vi "Volume ROI entry window.vi"(0 "Coordinates":i32[](array[numeric]), 1 "Do not initialise selector values":bool, 5 "AOLZ Settings":T1, 11 "ZplaneIndex (zero based)":i32, 12 "# of planes":i32) -> (4 "ROIs Info []":T2[](array[typedef]) {"FOV" min=1.0 max=10.0 step=1.0; "Frame Size" min=1.0 max=10.0 step=1.0; "Laser Power" min=1.0 max=10.0 step=0.10000000149011612; "Rel. Resolution" min=1.0 max=10.0 step=1.0; "POI Dwell time" min=1.0 max=10.0 step=0.10000000149011612; "Zoom" min=1.0 max=10.0 step=0.10000000149011612}, 10 "Zoom (out)":dbl=1.0 min=1.0 max=10.0 step=0.10000000149011612, 14 "Cancelled":bool)   [LabVIEW 2020]
uses:
  Typedefs/ROI spec.ctl
  Typedefs/ROI ID Enum.ctl
  ROI Entry screen/Typedefs/ROI Z-stack settings info.ctl
  ROI Entry screen/Typedefs/Volume entry ctrl refs cluster.ctl
  <vilib>/Utility/miscctls.llb/LVPointTypeDef.ctl
  ROI Entry screen/Globals/gl_Volume Entry UI globals.vi
  ROI Entry screen/Globals/gl_ROI Entry UI globals.vi
panel:
  in  "Laser Power (%)":dbl=1.0 min=0.001 max=10.0 step=0.10000000149011612
  in  "Rel. Resolution":dbl=1.0 min=0.001 max=10.0 step=0.10000000149011612
  in  "Dwell Time":dbl=1.0 min=0.001 max=10.0 step=0.10000000149011612
  in  "Z-step (planes)":i32=1 min=1 max=3 step=1
  in  "Dual Rectangle":bool
  in  "Zoom":dbl=1.0 min=0.001 max=10.0 step=0.10000000149011612
  in  "Cancel":bool
  in  "Proceed":bool
  in  "Z-plane 2":u16(ring) caption="Z-plane" items=["Z-plane 1", "Z-plane 2", "Z-plane 3", "Z-plane 4", "Z-plane 5", "Z-plane 6", "Z-plane 7", "Z-plane 8", "Z-plane 9", "Z-plane 10", "Z-plane 11"]
  in  "Z-plane 1":u16(ring) caption="Z-plane" items=["Z-plane 1", "Z-plane 2", "Z-plane 3", "Z-plane 4", "Z-plane 5", "Z-plane 6", "Z-plane 7", "Z-plane 8", "Z-plane 9", "Z-plane 10", "Z-plane 11"]
  in  "Volume":bool
  # "To specify a volume from the drawn rectangle, tick the Volume box and select the z-planes between which the volume should be generated.\n \nTo draw two rectangles at precisely the same XY position but on different z-levels, tick the \"Dual Rectangle\" box."
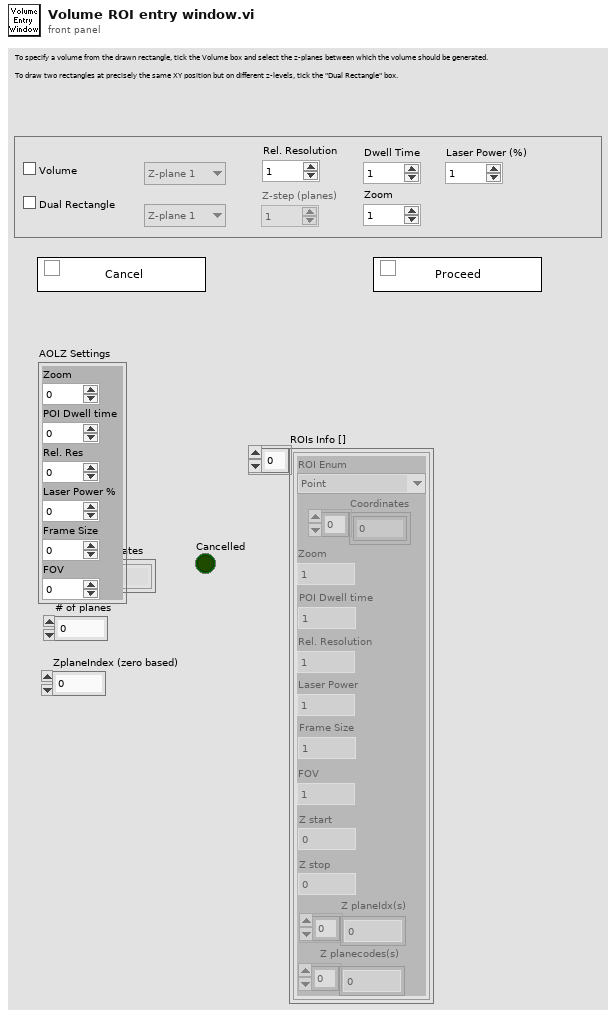
[diagram p1: front panel]
types:
  T1 = typedef "ROI Z-stack settings info.ctl" = cluster{"Zoom":dbl, "POI Dwell time":dbl, "Rel. Res":dbl, "Laser Power %":dbl, "Frame Size":dbl, "FOV":dbl}
  T2 = typedef "ROI spec.ctl" = cluster{"ROI Enum":T3, "Coordinates":i32[], "Zoom":dbl, "POI Dwell time":dbl, "Rel. Resolution":dbl, "Laser Power":dbl, "Frame Size":dbl, "FOV":dbl, "Z start":dbl, "Z stop":dbl, "Z planeIdx(s)":i32[], "Z planecodes(s)":u8[]}
  T3 = typedef "ROI ID Enum.ctl" = enum16{"Point", "MiniScan", "Comp. MiniScan", "Rectangle", "Comp. volume", "Arb. plane point", "None"}
  T4 = typedef "Volume entry ctrl refs cluster.ctl" = cluster{"Z-step (planes)":refnum<vi>, "Volume":refnum<vi>, "Dual Rectangle":refnum<vi>, "Zoom":refnum<vi>, "Z-plane 1":refnum<vi>, "Z-plane 2":refnum<vi>, "ZplaneIndex (zero based)":refnum<vi>}
  T5 = typedef "LVPointTypeDef.ctl" = cluster{"Horizontal":i16, "Vertical":i16}
  T6 = enum8{"Enabled", "Disabled", "Disabled and Grayed Out"}
  T7 = typedef "ROI input mode.ctl" = enum16{"Unspecified", "Point-Line-Plane", "Volume"}
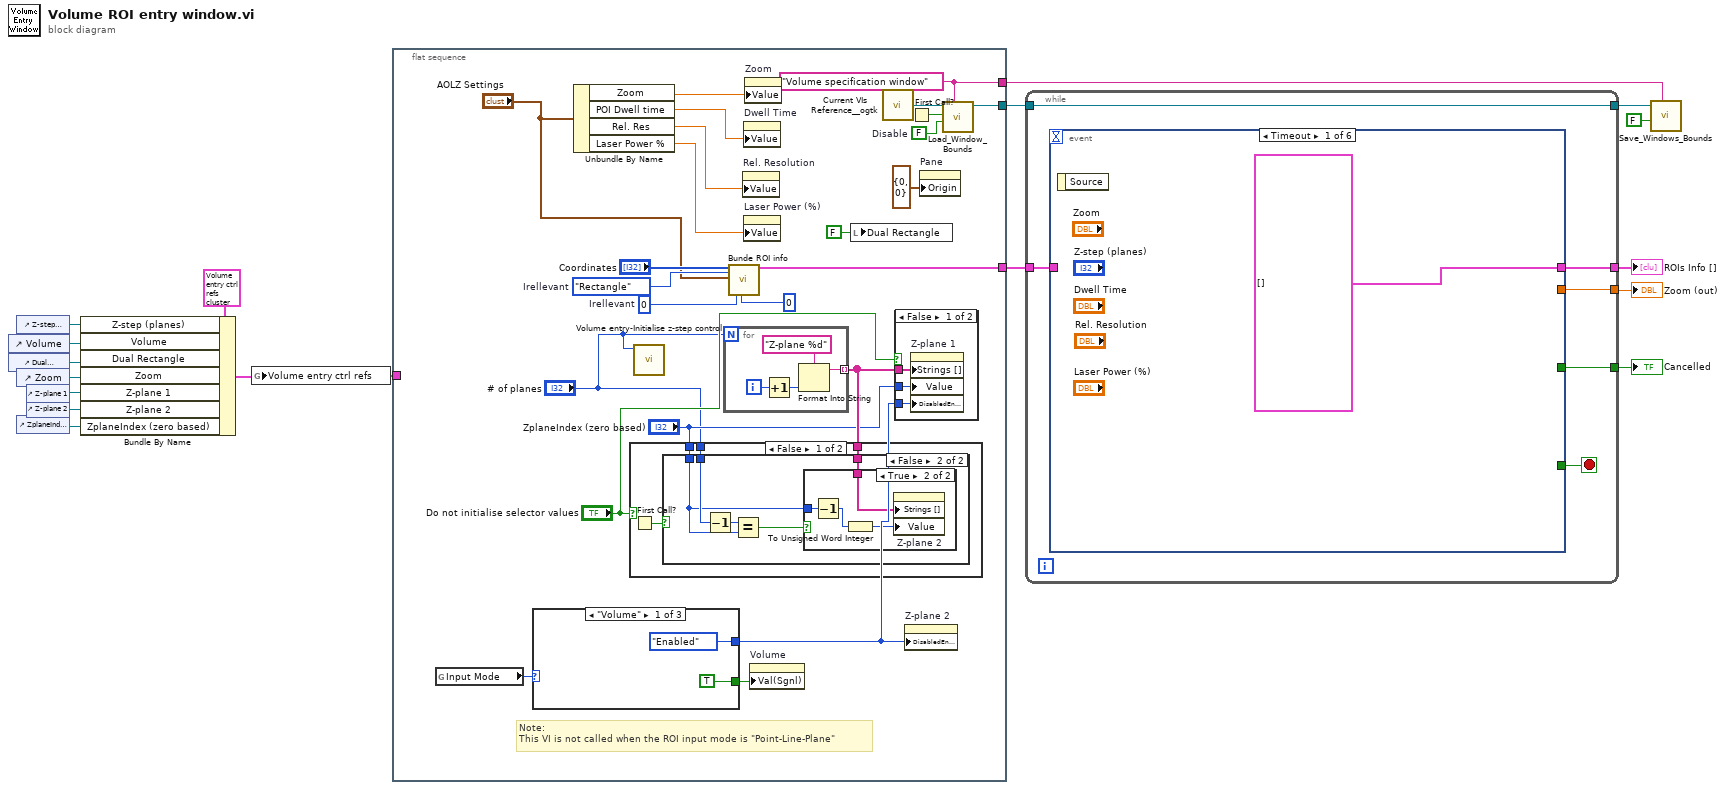
[diagram p0: block diagram]
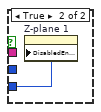
[diagram p2: hidden frame]
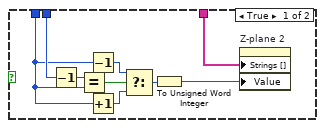
[diagram p3: hidden frame]
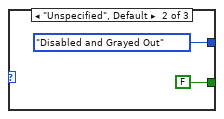
[diagram p6: hidden frame]
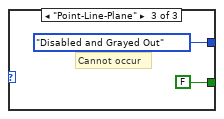
[diagram p7: hidden frame]
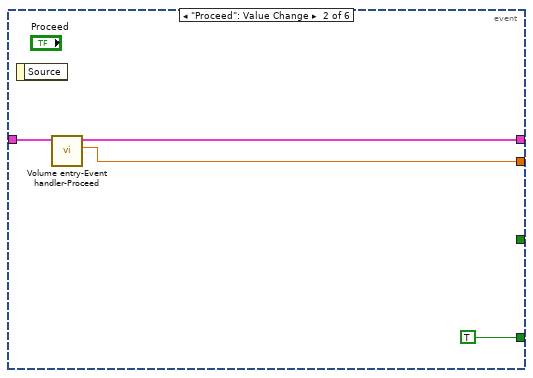
[diagram p8: hidden frame]
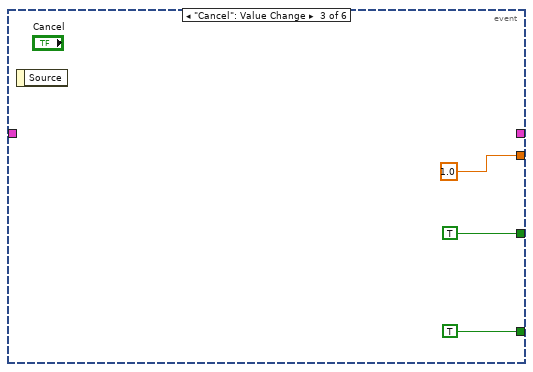
[diagram p9: hidden frame]
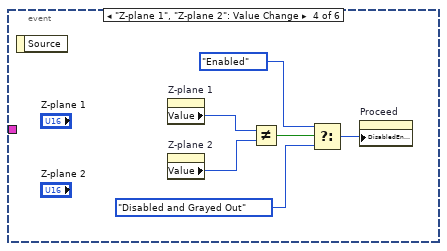
[diagram p10: hidden frame]
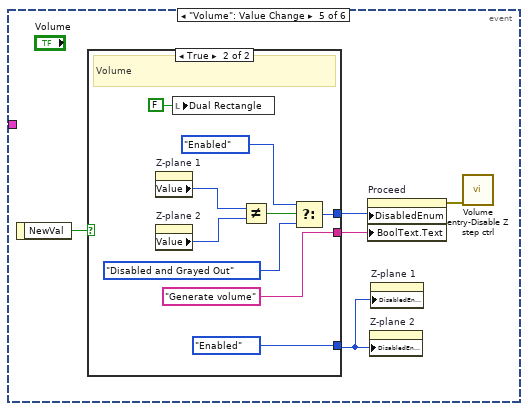
[diagram p11: hidden frame]
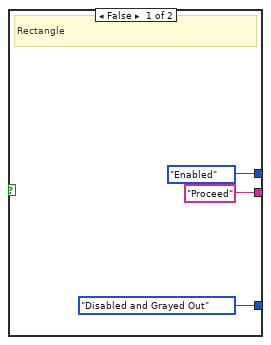
[diagram p12: hidden frame]
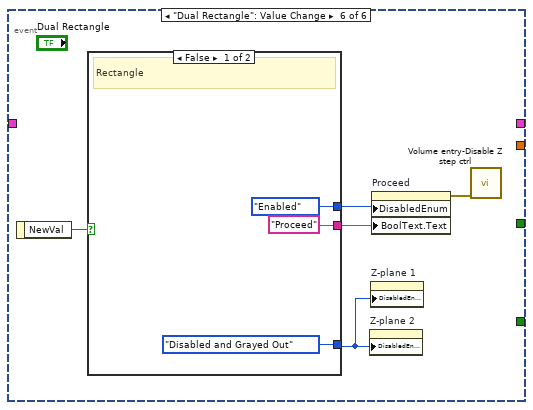
[diagram p13: hidden frame]
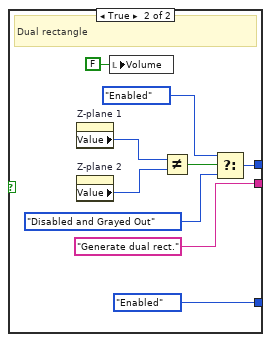
[diagram p14: hidden frame]
diagram:
  n1 = control-ref of="Volume"() -> (w6:refnum<vi>)
  n2 = control-ref of="Dual Rectangle"() -> (w5:refnum<vi>)
  n3 = control-ref of="Z-step (planes)"() -> (w8:refnum<vi>)
  n4 = control-ref of="Zoom"() -> (w4:refnum<vi>)
  n5 = control-ref of="ZplaneIndex (zero based)"() -> (w1:refnum<vi>)
  n6 = control-ref of="Z-plane 1"() -> (w3:refnum<vi>)
  n7 = control-ref of="Z-plane 2"() -> (w2:refnum<vi>)
  n8 = Bundle By Name(cluster=T4 {"Z-step (planes)"=refnum, "Volume"=refnum, "Dual Rectangle"=refnum, "Zoom"=refnum, "Z-plane 1"=refnum, "Z-plane 2"=refnum, "ZplaneIndex (zero based)"=refnum} ("Volume entry ctrl refs"), "Z-step (planes)"=w8, "Volume"=w6, "Dual Rectangle"=w5, "Zoom"=w4, "Z-plane 1"=w3, "Z-plane 2"=w2, "ZplaneIndex (zero based)"=w1) -> (w7:T4)
  n9 = global write "gl_Volume Entry UI globals.vi" "Volume entry ctrl refs"(w7) -> ()
  n10 = flat-sequence {
    tunnel: [w35] -> w15
    tunnel: [w31] -> w13
    tunnel: [w30] -> w11
    tunnel: w7 -> [_]
    frame #0 {
      w23 = 0  # Irellevant
      w29 = ROI_ID_Enum."Rectangle"  # Irellevant
      w32 = FALSE  # Disable
      w31 = "Volume specification window" ("Window Name (i.e. Key)")
      # "Note:\nThis VI is not called when the ROI input mode is \"Point-Line-Plane\""
      n11 = global read "gl_ROI Entry UI globals.vi" "Input Mode"() -> (w39:T7)
      n12 = case shown="\"Volume\"" w39 {
        tunnel: [TRUE ("Create Volume") FALSE ("Create Volume") FALSE ("Create Volume")] -> w38
        tunnel: [T6."Enabled" ("Disabled") T6."Disabled and Grayed Out" ("Disabled") T6."Disabled and Grayed Out" ("Disabled")] -> w26
        frame "Volume" {
        }
        frame "Unspecified", Default {
        }
        frame "Point-Line-Plane" {
          # "Cannot occur"
        }
      }
      n13 = Unbundle By Name("AOLZ Settings") -> ("Zoom"=w22:dbl, "POI Dwell time"=w21:dbl, "Rel. Res"=w20:dbl, "Laser Power %"=w19:dbl)
      n14 = call "Volume entry-Initialise z-step control.vi"("# of planes"="# of planes") -> ()  [unwired: 10 in, 1 out]
      n15 = for {
        N: "# of planes" -> [_]
        tunnel: [w75] -> w41 mode=indexing
        i -> [w77]
        n16 = Increment(x=w77) -> (x+1=w76:i32)
        n17 = Format Into String(format string="Z-plane %d", w76) -> (resulting string=w75:string)  [unwired: 2 in, 1 out]
      }
      n18 = case shown="False" "Do not initialise selector values" {
        tunnel: w41 -> [w49 _]
        tunnel: "# of planes" -> [w48 _]
        tunnel: "ZplaneIndex (zero based)" -> [w47 _]
        frame False {
          n19 = First Call?() -> (First Call?: T/F=w46:bool)
          n20 = case shown="False" w46 {
            tunnel: w49 -> [w58 w63]
            tunnel: w48 -> [w57 w62]
            tunnel: w47 -> [w50 w60]
            frame True {
              n21 = Decrement(x=w57) -> (x-1=w56:i32)
              n22 = Equal?(x=w56, y=w50) -> (x = y?=w55:bool)
              n23 = Decrement(x=w50) -> (x-1=w53:i32)
              n24 = Increment(x=w50) -> (x+1=w54:i32)
              n25 = Select(t=w53, s=w55, f=w54) -> (s? t:f=w52:i32)
              n26 = To Unsigned Word Integer(number=w52) -> (unsigned 16bit integer=w51:u16)
              n27 = property on="Z-plane 2" class="Ring (strict)"("Strings []"=w58, "Value"=w51) -> ()  [unwired: 2 in, 2 out]
            }
            frame False {
              n28 = Decrement(x=w62) -> (x-1=w61:i32)
              n29 = Equal?(x=w61, y=w60) -> (x = y?=w59:bool)
              n30 = case shown="True" w59 {
                tunnel: w63 -> [_ w67]
                tunnel: w60 -> [_ w65]
                frame False {
                }
                frame True {
                  n31 = Decrement(x=w65) -> (x-1=w64:i32)
                  n32 = To Unsigned Word Integer(number=w64) -> (unsigned 16bit integer=w66:u16)
                  n33 = property on="Z-plane 2" class="Ring (strict)"("Strings []"=w67, "Value"=w66) -> ()  [unwired: 2 in, 2 out]
                }
              }
            }
          }
        }
        frame True {
        }
      }
      n34 = call "Bunde ROI info.vi"("ROI Coordinates"="Coordinates", "ROI Enum"=w29, "Z stack Settings"="AOLZ Settings", "ZplaneIndex"=w23, "Zplanecode"=u8 0) -> ("ROI Info"=w35:T2)  [unwired: 14 in]
      n35 = property on="Rel. Resolution" class="DigNum (strict)"("Value"=w20) -> ()  [unwired: 2 in, 2 out]
      n36 = property on="Dwell Time" class="DigNum (strict)"("Value"=w21) -> ()  [unwired: 2 in, 2 out]
      n37 = property on="Laser Power (%)" class="DigNum (strict)"("Value"=w19) -> ()  [unwired: 2 in, 2 out]
      n38 = property on="Zoom" class="DigNum (strict)"("Value"=w22) -> ()  [unwired: 2 in, 2 out]
      n39 = property on="Volume" class="Bool (strict)"("Val(Sgnl)"=w38) -> ()  [unwired: 2 in, 2 out]
      n40 = local write "Dual Rectangle"(FALSE ("Dual Rectangle")) -> ()
      n41 = call <userlib>:"Current VIs Reference__ogtk.vi"() -> ("Current VI's reference"=w34:refnum<vi>)  [unwired: 5 in]
      n42 = case shown="False" "Do not initialise selector values" {
        tunnel: w41 -> [w44 _]
        tunnel: "ZplaneIndex (zero based)" -> [w43 _]
        tunnel: w26 -> [w42 w45]
        frame False {
          n43 = property on="Z-plane 1" class="Ring (strict)"("Strings []"=w44, "Value"=w43, "DisabledEnum"=w42) -> ()  [unwired: 2 in, 2 out]
        }
        frame True {
          n44 = property on="Z-plane 1" class="Ring (strict)"("DisabledEnum"=w45) -> ()  [unwired: 2 in, 2 out]
        }
      }
      n45 = property on="Z-plane 2" class="Ring (strict)"("DisabledEnum"=w26) -> ()  [unwired: 2 in, 2 out]
      n46 = First Call?() -> (First Call?: T/F=w33:bool)
      n47 = property on="Pane" class="Pane"("Origin"=T5 {"Horizontal"=0, "Vertical"=0}) -> ()  [unwired: 2 in, 2 out]
      n48 = call "Load_Window_Bounds.vi"("Window Name (i.e. Key)"=w31, "Disable"=w32, "First Call"=w33, "Window VI's Ref"=w34) -> ("reference out"=w30:refnum<vi>)  [unwired: 4 in, 3 out]
    }
  }
  n49 = while {
    tunnel: [w83] -> w17
    tunnel: w15 -> [w82]
    tunnel: [w80] -> w16
    tunnel: [w79] -> w14
    tunnel: w11 -> [w78]
    tunnel: [w78] -> w10
    stop <- w81 stop-if-true
    n50 = event shown="[0] Timeout" {
      selector: _ -> [_ _ _ _ _ _]
      dyn-events: _ -> [_ _ _ _ _ _]
      timeout: _ -> [_ _ _ _ _ _]
      tunnel: [T2[] [] ("ROIs Info []") w88 _ _ _ _] -> w83
      tunnel: w82 -> [_ w85 _ _ _ _]
      tunnel: [_ TRUE TRUE _ _ _] -> w81
      tunnel: [_ _ TRUE ("Cancel") _ _ _] -> w80
      tunnel: [_ w86 1.0 ("Zoom") _ _ _] -> w79
      event Timeout {
        n51 = event-data() -> ()  [unwired: 1 in, 1 out]
      }
      event "Proceed": Value Change {
        n52 = event-data() -> ()  [unwired: 1 in, 1 out]
        n53 = call "Volume entry-Event handler-Proceed.vi"("ROI Info"=w85) -> ("Zoom"=w86:dbl, "ROI Info []"=w88:T2[])  [unwired: 9 in]
      }
      event "Cancel": Value Change {
        n54 = event-data() -> ()  [unwired: 1 in, 1 out]
      }
      event "Z-plane 1", "Z-plane 2": Value Change {
        n55 = event-data() -> ()  [unwired: 1 in, 1 out]
        n56 = property on="Z-plane 1" class="Ring (strict)"() -> ("Value"=w97:u16)  [unwired: 2 in, 2 out]
        n57 = property on="Z-plane 2" class="Ring (strict)"() -> ("Value"=w96:u16)  [unwired: 2 in, 2 out]
        n58 = Not Equal?(x=w97, y=w96) -> (x != y?=w95:bool)
        n59 = Select(t=T6."Enabled" ("Disabled"), s=w95, f=T6."Disabled and Grayed Out" ("Disabled")) -> (s? t:f=w92:T6)
        n60 = property on="Proceed" class="Bool"("DisabledEnum"=w92) -> ()  [unwired: 2 in, 2 out]
      }
      event "Volume": Value Change {
        n61 = event-data() -> ("NewVal"=w101:bool)  [unwired: 1 in]
        n62 = case shown="True" w101 {
          tunnel: [T6."Enabled" ("Disabled") w109] -> w102
          tunnel: [T6."Disabled and Grayed Out" ("Disabled") T6."Enabled" ("Disabled")] -> w100
          tunnel: ["Proceed" "Generate volume"] -> w99
          frame False {
            # "Rectangle"
          }
          frame True {
            # "Volume"
            n63 = property on="Z-plane 1" class="Ring (strict)"() -> ("Value"=w114:u16)  [unwired: 2 in, 2 out]
            n64 = property on="Z-plane 2" class="Ring (strict)"() -> ("Value"=w113:u16)  [unwired: 2 in, 2 out]
            n65 = local write "Dual Rectangle"(FALSE ("Dual Rectangle")) -> ()
            n66 = Not Equal?(x=w114, y=w113) -> (x != y?=w112:bool)
            n67 = Select(t=T6."Enabled" ("Disabled"), s=w112, f=T6."Disabled and Grayed Out" ("Disabled")) -> (s? t:f=w109:T6)
          }
        }
        n68 = property on="Proceed" class="Bool"("DisabledEnum"=w102, "BoolText.Text"=w99) -> (error out=w98:errorcluster)  [unwired: 2 in, 1 out]
        n69 = property on="Z-plane 2" class="Ring (strict)"("DisabledEnum"=w100) -> ()  [unwired: 2 in, 2 out]
        n70 = property on="Z-plane 1" class="Ring (strict)"("DisabledEnum"=w100) -> ()  [unwired: 2 in, 2 out]
        n71 = call "Volume entry-Disable Z step ctrl.vi"("error in (no error)"=w98) -> ()  [unwired: 10 in, 1 out]
      }
      event "Dual Rectangle": Value Change {
        n72 = event-data() -> ("NewVal"=w117:bool)  [unwired: 1 in]
        n73 = case shown="False" w117 {
          tunnel: [T6."Enabled" ("Disabled") w126] -> w119
          tunnel: [T6."Disabled and Grayed Out" ("Disabled") T6."Enabled" ("Disabled")] -> w118
          tunnel: ["Proceed" "Generate dual rect."] -> w116
          frame False {
            # "Rectangle"
          }
          frame True {
            # "Dual rectangle"
            n74 = property on="Z-plane 1" class="Ring (strict)"() -> ("Value"=w131:u16)  [unwired: 2 in, 2 out]
            n75 = property on="Z-plane 2" class="Ring (strict)"() -> ("Value"=w130:u16)  [unwired: 2 in, 2 out]
            n76 = local write "Volume"(FALSE ("Volume")) -> ()
            n77 = Not Equal?(x=w131, y=w130) -> (x != y?=w129:bool)
            n78 = Select(t=T6."Enabled" ("Disabled"), s=w129, f=T6."Disabled and Grayed Out" ("Disabled")) -> (s? t:f=w126:T6)
          }
        }
        n79 = property on="Z-plane 2" class="Ring (strict)"("DisabledEnum"=w118) -> ()  [unwired: 2 in, 2 out]
        n80 = property on="Z-plane 1" class="Ring (strict)"("DisabledEnum"=w118) -> ()  [unwired: 2 in, 2 out]
        n81 = property on="Proceed" class="Bool"("DisabledEnum"=w119, "BoolText.Text"=w116) -> (error out=w115:errorcluster)  [unwired: 2 in, 1 out]
        n82 = call "Volume entry-Disable Z step ctrl.vi"("error in (no error)"=w115) -> ()  [unwired: 10 in, 1 out]
      }
    }
  }
  "ROIs Info []" <- w17
  "Cancelled" <- w16
  "Zoom (out)" <- w14
  n83 = call "Save_Windows_Bounds.vi"("Window Name (i.e. Key)"=w13, "Front Panel Window:Open"=FALSE, "Window VI's Ref"=w10) -> ()  [unwired: 8 in, 1 out]
